vi "LEP_RV_BuildSpec_UpdateUI.vi"(8 "error in (no error)":errorcluster, 9 "Build conflicts ref":refnum<vi>, 10 "Enable debugging ref":refnum<vi>, 11 "Action":enum16{"Init", "UpdateUI"}(ring)=enum."UpdateUI") -> (0 "error out":errorcluster)   [LabVIEW 2011]
uses:
  <vilib>/Platform/EmbProject/Plugins/utilities/LEP_Utilities_GetSetProjectData_U32.vi
  <vilib>/Platform/EmbProject/Plugins/utilities/LEP_Utilities_GetSetProjectData_I32.vi
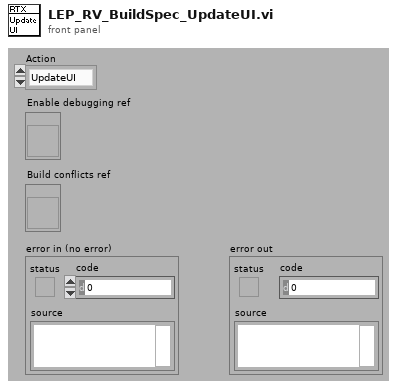
[diagram p1: front panel]
types:
  T1 = enum32{"Serial port", "TCP port", "USB ULINK2 JTAG"}
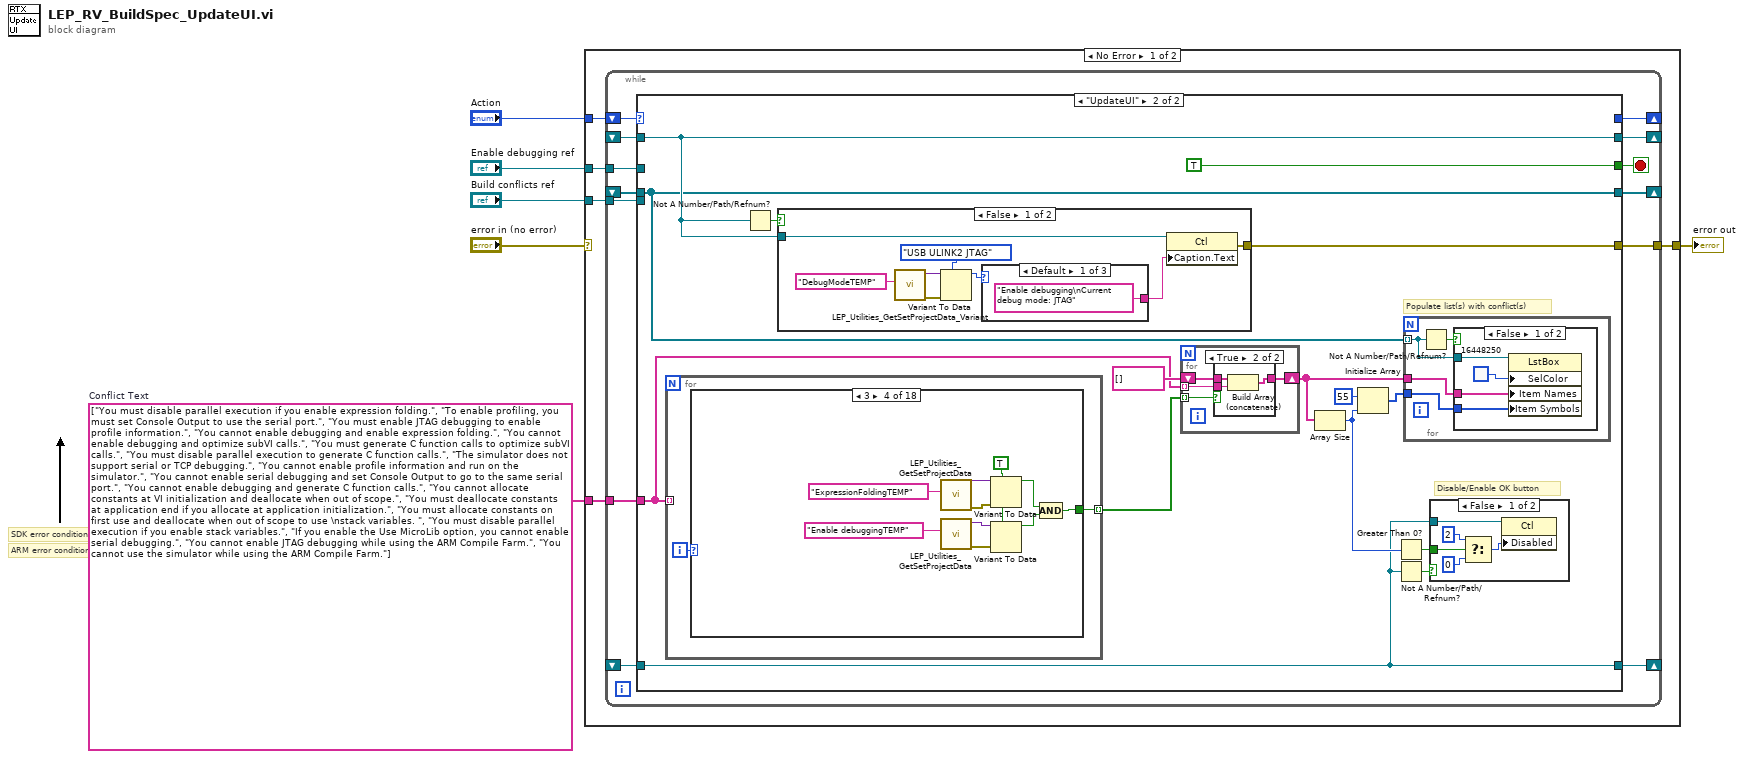
[diagram p0: block diagram]
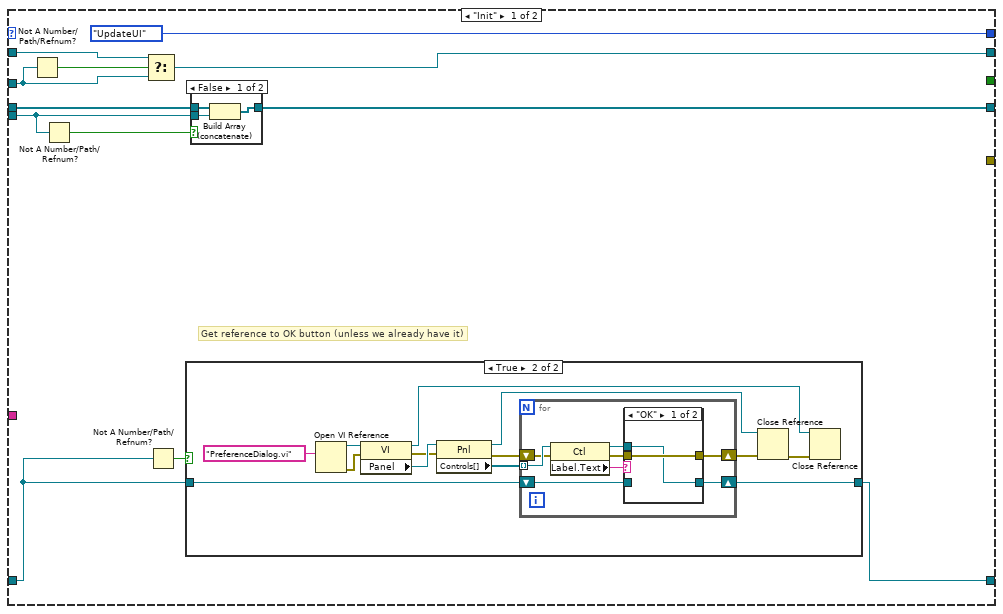
[diagram p2: hidden frame]
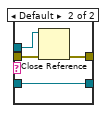
[diagram p4: hidden frame]
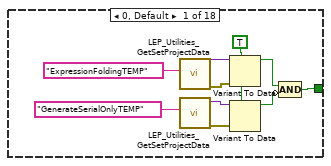
[diagram p9: hidden frame]
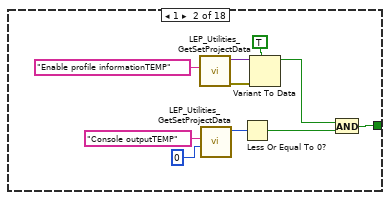
[diagram p10: hidden frame]
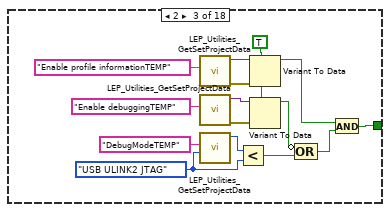
[diagram p11: hidden frame]
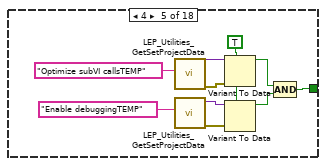
[diagram p12: hidden frame]
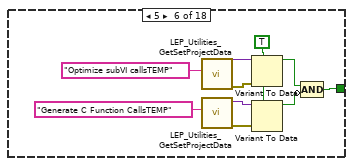
[diagram p13: hidden frame]
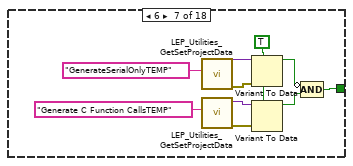
[diagram p14: hidden frame]
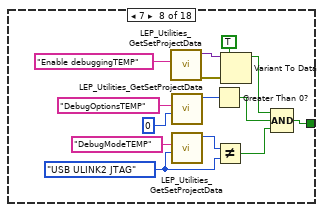
[diagram p15: hidden frame]
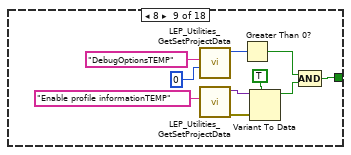
[diagram p16: hidden frame]
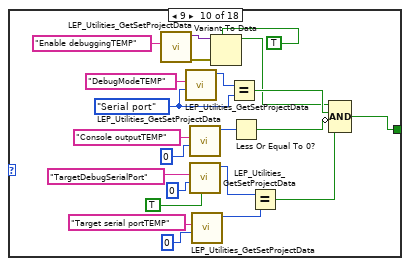
[diagram p17: hidden frame]
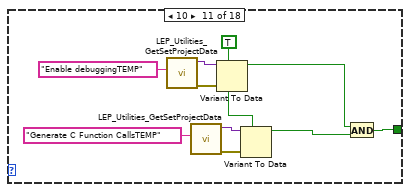
[diagram p18: hidden frame]
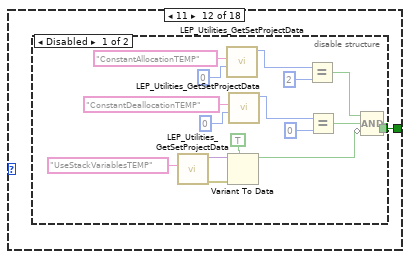
[diagram p19: hidden frame]
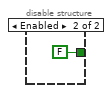
[diagram p20: hidden frame]
diagram:
  w1 = string[] ["You must disable parallel execution if you enable expression folding.", "To enable profiling, you must set Console Output to use the serial port.", "You must enable JTAG debugging to enable profile information.", "You cannot enable debugging and enable expression folding.", "You cannot enable debugging and optimize subVI calls.", "You must generate C function calls to optimize subVI calls.", "You must disable parallel execution to generate C function calls.", "The simulator does not support serial or TCP debugging.", "You cannot enable profile information and run on the simulator.", "You cannot enable serial debugging and set Console Output to go to the same serial port.", "You cannot enable debugging and generate C function calls.", "You cannot allocate constants at VI initialization and deallocate when out of scope.", "You must deallocate constants at application end if you allocate at application initialization.", "You must allocate constants on first use and deallocate when out of scope to use \nstack variables. ", "You must disable parallel execution if you enable stack variables.", "If you enable the Use MicroLib option, you cannot enable serial debugging.", "You cannot enable JTAG debugging while using the ARM Compile Farm.", "You cannot use the simulator while using the ARM Compile Farm."]  # Conflict Text
  # "ARM error conditions"
  # "SDK error conditions"
  n1 = case shown="No Error" "error in (no error)" {
    selector: "error in (no error)" -> [_ w347]
    tunnel: "Enable debugging ref" -> [w11 _]
    tunnel: "Action" -> [w10 _]
    tunnel: "Build conflicts ref" -> [w9 _]
    tunnel: [w8 w347] -> w2
    tunnel: w1 -> [w7 _]
    frame No Error {
      n2 = while {
        shift-right: [w22] -> _
        shift-left: _ -> [w24]
        tunnel: w11 -> [w23]
        shift-right: [w20] -> _
        shift-left: _ -> [w19]
        tunnel: w9 -> [w18]
        shift-right: [w17] -> _
        shift-left: w10 -> [w21]
        tunnel: [w16] -> w8
        tunnel: w7 -> [w14]
        shift-right: [w13] -> _
        shift-left: _ -> [w12]
        stop <- w15 stop-if-true
        n3 = case shown="\"UpdateUI\"" w21 {
          tunnel: w24 -> [w36 w82]
          tunnel: w23 -> [w35 _]
          tunnel: [w33 w82] -> w22
          tunnel: [w32 w79] -> w20
          tunnel: w19 -> [w31 w79]
          tunnel: w18 -> [w29 _]
          tunnel: [enum16{"Init", "UpdateUI"}."UpdateUI" ("Enum") _] -> w17
          tunnel: [_ w81] -> w16
          tunnel: [_ TRUE] -> w15
          tunnel: w14 -> [_ w77]
          tunnel: [w27 w71] -> w13
          tunnel: w12 -> [w25 w71]
          frame "Init" {
            # "Get reference to OK button (unless we already have it)"
            n4 = Not A Number/Path/Refnum?(number/path/refnum=w35) -> (NaN/Path/Refnum?=w34:bool)
            n5 = Not A Number/Path/Refnum?(number/path/refnum=w29) -> (NaN/Path/Refnum?=w28:bool)
            n6 = Select(t=w36, s=w34, f=w35) -> (s? t:f=w33:refnum<vi>)
            n7 = Not A Number/Path/Refnum?(number/path/refnum=w25) -> (NaN/Path/Refnum?=w26:bool)
            n8 = case shown="True" w26 {
              tunnel: [w37 w39] -> w27
              tunnel: w25 -> [w37 w38]
              frame False {
              }
              frame True {
                n9 = Open VI Reference(vi path="PreferenceDialog.vi") -> (vi reference=w48:refnum<vi>, error out=w49:errorcluster)  [unwired: 1 in, 4 out]
                n10 = property class="VI"(reference=w48, error in=w49) -> (reference out=w40:refnum<vi>, error out=w46:errorcluster, "Panel"=w47:refnum<vi>)
                n11 = property class="Pnl"(reference=w47, error in=w46) -> (reference out=w41:refnum<vi>, error out=w44:errorcluster, "Controls[]"=w45:refnum<vi>[])
                n12 = for {
                  tunnel: w45 -> [w58] mode=indexing
                  shift-right: [w55] -> w43
                  shift-left: w44 -> [w57]
                  shift-right: [w52] -> w39
                  shift-left: w38 -> [w51]
                  n13 = property class="Ctl"(reference=w58, error in=w57) -> (reference out=w54:refnum<vi>, error out=w56:errorcluster, "Label.Text"=w53:string)
                  n14 = case shown="\"OK\"" w53 {
                    tunnel: w56 -> [w60 w64]
                    tunnel: [w60 w63] -> w55
                    tunnel: w54 -> [w59 w62]
                    tunnel: [w59 w61] -> w52
                    tunnel: w51 -> [_ w61]
                    frame "OK" {
                    }
                    frame Default {
                      n15 = Close Reference(reference=w62, error in (no error)=w64) -> (error out=w63:errorcluster)
                    }
                  }
                }
                n16 = Close Reference(reference=w41, error in (no error)=w43) -> (error out=w42:errorcluster)
                n17 = Close Reference(reference=w40, error in (no error)=w42) -> ()  [unwired: 1 out]
              }
            }
            n18 = case shown="False" w28 {
              tunnel: [w67 w68] -> w32
              tunnel: w29 -> [w66 _]
              tunnel: w31 -> [w65 w68]
              frame False {
                n19 = Build Array (concatenate)(w65, w66) -> (w67:refnum<vi>[])
              }
              frame True {
              }
            }
          }
          frame "UpdateUI" {
            # "Populate list(s) with conflict(s)"
            # "Disable/Enable OK button"
            n20 = for {
              tunnel: w77 -> [_] mode=indexing
              tunnel: [w105] -> w70 mode=indexing
              i -> [w106]
              n21 = case shown="3" w106 {
                tunnel: [w108 w120 w130 w142 w152 w162 w172 w193 w203 w219 w231 w238 w256 w274 w294 w310 w326 w335] -> w105
                frame 0, Default {
                  w107 = TRUE
                  n22 = call-poly <vilib>:"LEP_Utilities_GetSetProjectData.vi"("ItemName"="ExpressionFoldingTEMP") -> ("error out"=w112:errorcluster, "Variant Out"=w113:variant)  [unwired: 4 in, 5 out]
                  n23 = call-poly <vilib>:"LEP_Utilities_GetSetProjectData.vi"("ItemName"="GenerateSerialOnlyTEMP") -> ("error out"=w114:errorcluster, "Variant Out"=w115:variant)  [unwired: 4 in, 5 out]
                  n24 = Variant To Data(error in=w112, type=w107, Variant=w113) -> (data=w116:bool)  [unwired: 1 out]
                  n25 = Variant To Data(error in=w114, type=w107, Variant=w115) -> (data=w109:bool)  [unwired: 1 out]
                  n26 = Compound Arithmetic op=AND(w116, invert w109) -> (w108:bool)
                }
                frame 1 {
                  n27 = call-poly <vilib>:"LEP_Utilities_GetSetProjectData.vi"("ItemName"="Enable profile informationTEMP") -> ("error out"=w122:errorcluster, "Variant Out"=w123:variant)  [unwired: 4 in, 5 out]
                  n28 = call-poly <vilib>:"LEP_Utilities_GetSetProjectData.vi"("data in"=u32 0, "ItemName"="Console outputTEMP") -> ("data out"=w118:u32)  [unwired: 3 in, 6 out]
                  n29 = Less Or Equal To 0?(x=w118) -> (x <= 0?=w117:bool)
                  n30 = Variant To Data(error in=w122, type=TRUE, Variant=w123) -> (data=w124:bool)  [unwired: 1 out]
                  n31 = And(x=w124, y=w117) -> (x .and. y?=w120:bool)
                }
                frame 2 {
                  w128 = T1."USB ULINK2 JTAG" ("Debugging mode")
                  w141 = TRUE
                  n32 = call-poly <vilib>:"LEP_Utilities_GetSetProjectData.vi"("ItemName"="Enable profile informationTEMP") -> ("error out"=w134:errorcluster, "Variant Out"=w135:variant)  [unwired: 4 in, 5 out]
                  n33 = call-poly <vilib>:"LEP_Utilities_GetSetProjectData.vi"("ItemName"="Enable debuggingTEMP") -> ("error out"=w136:errorcluster, "Variant Out"=w137:variant)  [unwired: 4 in, 5 out]
                  n34 = call-poly <vilib>:"LEP_Utilities_GetSetProjectData.vi"("data in"=w128, "ItemName"="DebugModeTEMP") -> ("data out"=w129:u32)  [unwired: 3 in, 6 out]
                  n35 = Less?(x=w129, y=w128) -> (x < y?=w127:bool)
                  n36 = Variant To Data(error in=w134, type=w141, Variant=w135) -> (data=w138:bool)  [unwired: 1 out]
                  n37 = Variant To Data(error in=w136, type=w141, Variant=w137) -> (data=w131:bool)  [unwired: 1 out]
                  n38 = Compound Arithmetic op=OR(invert w131, w127) -> (w139:bool)
                  n39 = And(x=w138, y=w139) -> (x .and. y?=w130:bool)
                }
                frame 3 {
                  w149 = TRUE
                  n40 = call-poly <vilib>:"LEP_Utilities_GetSetProjectData.vi"("ItemName"="ExpressionFoldingTEMP") -> ("error out"=w145:errorcluster, "Variant Out"=w146:variant)  [unwired: 4 in, 5 out]
                  n41 = call-poly <vilib>:"LEP_Utilities_GetSetProjectData.vi"("ItemName"="Enable debuggingTEMP") -> ("error out"=w147:errorcluster, "Variant Out"=w148:variant)  [unwired: 4 in, 5 out]
                  n42 = Variant To Data(error in=w145, type=w149, Variant=w146) -> (data=w150:bool)  [unwired: 1 out]
                  n43 = Variant To Data(error in=w147, type=w149, Variant=w148) -> (data=w151:bool)  [unwired: 1 out]
                  n44 = Compound Arithmetic op=AND(w150, w151) -> (w142:bool)
                }
                frame 4 {
                  w159 = TRUE
                  n45 = call-poly <vilib>:"LEP_Utilities_GetSetProjectData.vi"("ItemName"="Optimize subVI callsTEMP") -> ("error out"=w155:errorcluster, "Variant Out"=w156:variant)  [unwired: 4 in, 5 out]
                  n46 = call-poly <vilib>:"LEP_Utilities_GetSetProjectData.vi"("ItemName"="Enable debuggingTEMP") -> ("error out"=w157:errorcluster, "Variant Out"=w158:variant)  [unwired: 4 in, 5 out]
                  n47 = Variant To Data(error in=w155, type=w159, Variant=w156) -> (data=w160:bool)  [unwired: 1 out]
                  n48 = Variant To Data(error in=w157, type=w159, Variant=w158) -> (data=w161:bool)  [unwired: 1 out]
                  n49 = Compound Arithmetic op=AND(w160, w161) -> (w152:bool)
                }
                frame 5 {
                  w169 = TRUE
                  n50 = call-poly <vilib>:"LEP_Utilities_GetSetProjectData.vi"("ItemName"="Optimize subVI callsTEMP") -> ("error out"=w165:errorcluster, "Variant Out"=w166:variant)  [unwired: 4 in, 5 out]
                  n51 = call-poly <vilib>:"LEP_Utilities_GetSetProjectData.vi"("ItemName"="Generate C Function CallsTEMP") -> ("error out"=w167:errorcluster, "Variant Out"=w168:variant)  [unwired: 4 in, 5 out]
                  n52 = Variant To Data(error in=w165, type=w169, Variant=w166) -> (data=w170:bool)  [unwired: 1 out]
                  n53 = Variant To Data(error in=w167, type=w169, Variant=w168) -> (data=w171:bool)  [unwired: 1 out]
                  n54 = Compound Arithmetic op=AND(w170, invert w171) -> (w162:bool)
                }
                frame 6 {
                  w179 = TRUE
                  n55 = call-poly <vilib>:"LEP_Utilities_GetSetProjectData.vi"("ItemName"="GenerateSerialOnlyTEMP") -> ("error out"=w175:errorcluster, "Variant Out"=w176:variant)  [unwired: 4 in, 5 out]
                  n56 = call-poly <vilib>:"LEP_Utilities_GetSetProjectData.vi"("ItemName"="Generate C Function CallsTEMP") -> ("error out"=w177:errorcluster, "Variant Out"=w178:variant)  [unwired: 4 in, 5 out]
                  n57 = Variant To Data(error in=w175, type=w179, Variant=w176) -> (data=w180:bool)  [unwired: 1 out]
                  n58 = Variant To Data(error in=w177, type=w179, Variant=w178) -> (data=w181:bool)  [unwired: 1 out]
                  n59 = Compound Arithmetic op=AND(invert w180, w181) -> (w172:bool)
                }
                frame 7 {
                  w191 = T1."USB ULINK2 JTAG" ("Debugging mode")
                  n60 = call-poly <vilib>:"LEP_Utilities_GetSetProjectData.vi"("ItemName"="Enable debuggingTEMP") -> ("error out"=w185:errorcluster, "Variant Out"=w186:variant)  [unwired: 4 in, 5 out]
                  n61 = call-poly <vilib>:"LEP_Utilities_GetSetProjectData.vi"("data in"=u32 0, "ItemName"="DebugOptionsTEMP") -> ("data out"=w188:u32)  [unwired: 3 in, 6 out]
                  n62 = call-poly <vilib>:"LEP_Utilities_GetSetProjectData.vi"("data in"=w191, "ItemName"="DebugModeTEMP") -> ("data out"=w192:u32)  [unwired: 3 in, 6 out]
                  n63 = Greater Than 0?(x=w188) -> (x > 0?=w187:bool)
                  n64 = Not Equal?(x=w192, y=w191) -> (x != y?=w189:bool)
                  n65 = Variant To Data(error in=w185, type=TRUE, Variant=w186) -> (data=w182:bool)  [unwired: 1 out]
                  n66 = Compound Arithmetic op=AND(w182, w187, w189) -> (w193:bool)
                }
                frame 8 {
                  n67 = call-poly <vilib>:"LEP_Utilities_GetSetProjectData.vi"("data in"=u32 0, "ItemName"="DebugOptionsTEMP") -> ("data out"=w201:u32)  [unwired: 3 in, 6 out]
                  n68 = call-poly <vilib>:"LEP_Utilities_GetSetProjectData.vi"("ItemName"="Enable profile informationTEMP") -> ("error out"=w198:errorcluster, "Variant Out"=w197:variant)  [unwired: 4 in, 5 out]
                  n69 = Greater Than 0?(x=w201) -> (x > 0?=w200:bool)
                  n70 = Variant To Data(error in=w198, type=TRUE, Variant=w197) -> (data=w196:bool)  [unwired: 1 out]
                  n71 = Compound Arithmetic op=AND(w200, w196) -> (w203:bool)
                }
                frame 9 {
                  w223 = T1."Serial port" ("Debugging mode")
                  n72 = call-poly <vilib>:"LEP_Utilities_GetSetProjectData.vi"("ItemName"="Enable debuggingTEMP") -> ("error out"=w218:errorcluster, "Variant Out"=w214:variant)  [unwired: 4 in, 5 out]
                  n73 = call-poly <vilib>:"LEP_Utilities_GetSetProjectData.vi"("data in"=w223, "ItemName"="DebugModeTEMP") -> ("data out"=w222:u32)  [unwired: 3 in, 6 out]
                  n74 = call-poly <vilib>:"LEP_Utilities_GetSetProjectData.vi"("data in"=u32 0, "ItemName"="Console outputTEMP") -> ("data out"=w225:u32)  [unwired: 3 in, 6 out]
                  n75 = call-poly <vilib>:"LEP_Utilities_GetSetProjectData.vi"("access target data (F)"=TRUE, "data in"=0, "ItemName"="TargetDebugSerialPort") -> ("data out"=w212:i32)  [unwired: 2 in, 6 out]
                  n76 = call-poly <vilib>:"LEP_Utilities_GetSetProjectData.vi"("data in"=0, "ItemName"="Target serial portTEMP") -> ("data out"=w207:i32)  [unwired: 3 in, 6 out]
                  n77 = Variant To Data(error in=w218, type=TRUE, Variant=w214) -> (data=w215:bool)  [unwired: 1 out]
                  n78 = Equal?(x=w222, y=w223) -> (x = y?=w220:bool)
                  n79 = Less Or Equal To 0?(x=w225) -> (x <= 0?=w221:bool)
                  n80 = Equal?(x=w212, y=w207) -> (x = y?=w211:bool)
                  n81 = Compound Arithmetic op=AND(w215, w220, invert w221, w211) -> (w219:bool)
                }
                frame 10 {
                  w228 = TRUE
                  n82 = call-poly <vilib>:"LEP_Utilities_GetSetProjectData.vi"("ItemName"="Enable debuggingTEMP") -> ("error out"=w237:errorcluster, "Variant Out"=w235:variant)  [unwired: 4 in, 5 out]
                  n83 = call-poly <vilib>:"LEP_Utilities_GetSetProjectData.vi"("ItemName"="Generate C Function CallsTEMP") -> ("error out"=w233:errorcluster, "Variant Out"=w234:variant)  [unwired: 4 in, 5 out]
                  n84 = Variant To Data(error in=w237, type=w228, Variant=w235) -> (data=w230:bool)  [unwired: 1 out]
                  n85 = Variant To Data(error in=w233, type=w228, Variant=w234) -> (data=w229:bool)  [unwired: 1 out]
                  n86 = And(x=w230, y=w229) -> (x .and. y?=w231:bool)
                }
                frame 11 {
                  n87 = disable-structure shown="Disabled" {
                    disable-tunnel: [w248 FALSE] -> w238
                    frame Disabled {
                      n88 = call-poly <vilib>:"LEP_Utilities_GetSetProjectData.vi"("ItemName"="UseStackVariablesTEMP") -> ("error out"=w241:errorcluster, "Variant Out"=w242:variant)  [unwired: 4 in, 5 out]
                      n89 = call-poly <vilib>:"LEP_Utilities_GetSetProjectData.vi"("data in"=u32 0, "ItemName"="ConstantAllocationTEMP") -> ("data out"=w249:u32)  [unwired: 3 in, 6 out]
                      n90 = Variant To Data(error in=w241, type=TRUE, Variant=w242) -> (data=w239:bool)  [unwired: 1 out]
                      n91 = call-poly <vilib>:"LEP_Utilities_GetSetProjectData.vi"("data in"=u32 0, "ItemName"="ConstantDeallocationTEMP") -> ("data out"=w250:u32)  [unwired: 3 in, 6 out]
                      n92 = Equal?(x=w249, y=u32 2) -> (x = y?=w246:bool)
                      n93 = Equal?(x=w250, y=u32 0) -> (x = y?=w247:bool)
                      n94 = Compound Arithmetic op=AND(w246, w247, invert w239) -> (w248:bool)
                    }
                    frame Enabled {
                    }
                  }
                }
                frame 12 {
                  n95 = disable-structure shown="Disabled" {
                    disable-tunnel: [w266 FALSE] -> w256
                    frame Disabled {
                      n96 = call-poly <vilib>:"LEP_Utilities_GetSetProjectData.vi"("ItemName"="UseStackVariablesTEMP") -> ("error out"=w259:errorcluster, "Variant Out"=w260:variant)  [unwired: 4 in, 5 out]
                      n97 = call-poly <vilib>:"LEP_Utilities_GetSetProjectData.vi"("data in"=u32 0, "ItemName"="ConstantAllocationTEMP") -> ("data out"=w268:u32)  [unwired: 3 in, 6 out]
                      n98 = call-poly <vilib>:"LEP_Utilities_GetSetProjectData.vi"("data in"=u32 0, "ItemName"="ConstantDeallocationTEMP") -> ("data out"=w264:u32)  [unwired: 3 in, 6 out]
                      n99 = Variant To Data(error in=w259, type=TRUE, Variant=w260) -> (data=w257:bool)  [unwired: 1 out]
                      n100 = Equal?(x=w268, y=u32 3) -> (x = y?=w265:bool)
                      n101 = Not Equal?(x=w264, y=u32 2) -> (x != y?=w262:bool)
                      n102 = Compound Arithmetic op=AND(w265, w262, invert w257) -> (w266:bool)
                    }
                    frame Enabled {
                    }
                  }
                }
                frame 13 {
                  n103 = disable-structure shown="Disabled" {
                    disable-tunnel: [w279 FALSE] -> w274
                    frame Disabled {
                      n104 = call-poly <vilib>:"LEP_Utilities_GetSetProjectData.vi"("ItemName"="UseStackVariablesTEMP") -> ("error out"=w290:errorcluster, "Variant Out"=w289:variant)  [unwired: 4 in, 5 out]
                      n105 = call-poly <vilib>:"LEP_Utilities_GetSetProjectData.vi"("data in"=u32 0, "ItemName"="ConstantAllocationTEMP") -> ("data out"=w283:u32)  [unwired: 3 in, 6 out]
                      n106 = call-poly <vilib>:"LEP_Utilities_GetSetProjectData.vi"("data in"=u32 0, "ItemName"="ConstantDeallocationTEMP") -> ("data out"=w282:u32)  [unwired: 3 in, 6 out]
                      n107 = Variant To Data(error in=w290, type=TRUE, Variant=w289) -> (data=w275:bool)  [unwired: 1 out]
                      n108 = Not Equal?(x=w283, y=u32 0) -> (x != y?=w276:bool)
                      n109 = Not Equal?(x=w282, y=u32 0) -> (x != y?=w277:bool)
                      n110 = Or(x=w276, y=w277) -> (x .or. y?=w278:bool)
                      n111 = And(x=w275, y=w278) -> (x .and. y?=w279:bool)
                    }
                    frame Enabled {
                    }
                  }
                }
                frame 14 {
                  n112 = call-poly <vilib>:"LEP_Utilities_GetSetProjectData.vi"("ItemName"="GenerateSerialOnlyTEMP") -> ("error out"=w302:errorcluster, "Variant Out"=w293:variant)  [unwired: 4 in, 5 out]
                  n113 = call-poly <vilib>:"LEP_Utilities_GetSetProjectData.vi"("ItemName"="UseStackVariablesTEMP") -> ("error out"=w300:errorcluster, "Variant Out"=w301:variant)  [unwired: 4 in, 5 out]
                  n114 = Variant To Data(error in=w302, type=TRUE, Variant=w293) -> (data=w295:bool)  [unwired: 1 out]
                  n115 = Variant To Data(error in=w300, type=TRUE, Variant=w301) -> (data=w296:bool)  [unwired: 1 out]
                  n116 = Compound Arithmetic op=AND(w296, invert w295) -> (w294:bool)
                }
                frame 15 {
                  w305 = TRUE
                  w313 = T1."TCP port" ("Debugging mode")
                  n117 = call-poly <vilib>:"LEP_Utilities_GetSetProjectData.vi"("ItemName"="Use MicroLibTEMP") -> ("error out"=w307:errorcluster, "Variant Out"=w306:variant)  [unwired: 4 in, 5 out]
                  n118 = call-poly <vilib>:"LEP_Utilities_GetSetProjectData.vi"("ItemName"="Enable debuggingTEMP") -> ("error out"=w316:errorcluster, "Variant Out"=w317:variant)  [unwired: 4 in, 5 out]
                  n119 = call-poly <vilib>:"LEP_Utilities_GetSetProjectData.vi"("data in"=w313, "ItemName"="DebugModeTEMP") -> ("data out"=w314:u32)  [unwired: 3 in, 6 out]
                  n120 = Less?(x=w314, y=w313) -> (x < y?=w312:bool)
                  n121 = Variant To Data(error in=w307, type=w305, Variant=w306) -> (data=w304:bool)  [unwired: 1 out]
                  n122 = Variant To Data(error in=w316, type=w305, Variant=w317) -> (data=w311:bool)  [unwired: 1 out]
                  n123 = Compound Arithmetic op=AND(w311, w312) -> (w309:bool)
                  n124 = And(x=w304, y=w309) -> (x .and. y?=w310:bool)
                }
                frame 16 {
                  w328 = T1."USB ULINK2 JTAG" ("Debugging mode")
                  n125 = call "LEP_RV_LaunchLoadConfig.vi"() -> ("Connect to a network compile server"=w319:bool)  [unwired: 8 in, 7 out]
                  n126 = call-poly <vilib>:"LEP_Utilities_GetSetProjectData.vi"("data in"=w328, "ItemName"="DebugModeTEMP") -> ("data out"=w327:u32)  [unwired: 3 in, 6 out]
                  n127 = call-poly <vilib>:"LEP_Utilities_GetSetProjectData.vi"("ItemName"="Enable debuggingTEMP") -> ("error out"=w323:errorcluster, "Variant Out"=w324:variant)  [unwired: 4 in, 5 out]
                  n128 = Equal?(x=w327, y=w328) -> (x = y?=w325:bool)
                  n129 = Variant To Data(error in=w323, type=TRUE, Variant=w324) -> (data=w320:bool)  [unwired: 1 out]
                  n130 = Compound Arithmetic op=AND(w319, w325, w320) -> (w326:bool)
                }
                frame 17 {
                  n131 = call "LEP_RV_LaunchLoadConfig.vi"() -> ("Connect to a network compile server"=w334:bool)  [unwired: 8 in, 7 out]
                  n132 = call-poly <vilib>:"LEP_Utilities_GetSetProjectData.vi"("data in"=u32 0, "ItemName"="DebugOptionsTEMP") -> ("data out"=w331:u32)  [unwired: 3 in, 6 out]
                  n133 = Greater Than 0?(x=w331) -> (x > 0?=w330:bool)
                  n134 = And(x=w334, y=w330) -> (x .and. y?=w335:bool)
                }
              }
            }
            n135 = Not A Number/Path/Refnum?(number/path/refnum=w82) -> (NaN/Path/Refnum?=w83:bool)
            n136 = case shown="False" w83 {
              tunnel: w82 -> [w343 _]
              tunnel: [w342 _] -> w81
              frame False {
                n137 = call <vilib>:"LEP_Utilities_GetSetProjectData_Variant.vi"("ItemName"="DebugModeTEMP") -> ("error out"=w337:errorcluster, "Variant Out"=w338:variant)  [unwired: 4 in, 5 out]
                n138 = Variant To Data(error in=w337, type=T1."USB ULINK2 JTAG" ("Debugging mode"), Variant=w338) -> (data=w341:T1)  [unwired: 1 out]
                n139 = case shown="Default" w341 {
                  tunnel: ["Enable debugging\nCurrent debug mode: JTAG" "Enable debugging\nCurrent debug mode: Serial" "Enable debugging\nCurrent debug mode: TCP"] -> w340
                  frame Default {
                  }
                  frame "Serial port" {
                  }
                  frame "TCP port" {
                  }
                }
                n140 = property class="Ctl"(reference=w343, "Caption.Text"=w340) -> (error out=w342:errorcluster)  [unwired: 1 in, 1 out]
              }
              frame True {
              }
            }
            n141 = for {
              shift-right: [w89] -> w75
              shift-left: string[] [] -> [w92]
              tunnel: w70 -> [w91] mode=indexing
              tunnel: w77 -> [w90] mode=indexing
              n142 = case shown="True" w91 {
                tunnel: w92 -> [w93 w96]
                tunnel: w90 -> [_ w95]
                tunnel: [w93 w94] -> w89
                frame False {
                }
                frame True {
                  n143 = Build Array (concatenate)(w96, w95) -> (w94:string[])
                }
              }
            }
            n144 = Array Size(array=w75) -> (size(s)=w74:i32)
            n145 = Initialize Array(55, w74) -> (w69:i32[])
            n146 = Greater Than 0?(x=w74) -> (x > 0?=w72:bool)
            n147 = Not A Number/Path/Refnum?(number/path/refnum=w71) -> (NaN/Path/Refnum?=w73:bool)
            n148 = for {
              tunnel: w79 -> [w99] mode=indexing
              tunnel: w69 -> [w98]
              tunnel: w75 -> [w97]
              n149 = Not A Number/Path/Refnum?(number/path/refnum=w99) -> (NaN/Path/Refnum?=w100:bool)
              n150 = case shown="False" w100 {
                tunnel: w99 -> [w104 _]
                tunnel: w98 -> [w103 _]
                tunnel: w97 -> [w102 _]
                frame False {
                  n151 = property class="LstBox"(reference=w104, "SelColor"=u32 16448250, "Item Names"=w102, "Item Symbols"=w103) -> ()  [unwired: 1 in, 2 out]
                }
                frame True {
                }
              }
            }
            n152 = case shown="False" w73 {
              tunnel: w72 -> [w88 _]
              tunnel: w71 -> [w87 _]
              frame False {
                n153 = Select(t=u8 2 ("Disabled"), s=w88, f=u8 0) -> (s? t:f=w86:u8)
                n154 = property class="Ctl"(reference=w87, "Disabled"=w86) -> ()  [unwired: 1 in, 2 out]
              }
              frame True {
              }
            }
          }
        }
      }
    }
    frame Error {
    }
  }
  "error out" <- w2
